vi "Coeficientes do polinômio.vi"(1 "R":dbl=0.06009682, 2 "Infos para processamento":T1={"Diâmetro do furo [mm]"=1.4, "Diâmetro da linha média [mm]"=5.0, "IncF"=0.2, "Módulo de elasticidade [GPa]"=207.0, "Módulo de Poisson"=0.3, "Tipo de roseta utilizada"=enum."Tipo A", "Método de análise"=enum."Simplificado 2008", "Pfinal"=0.3, "Parar auto."=TRUE}, 3 "Resultados":dbl[][](array[numeric])) -> (0 "Coeficientes":dbl[][](array[numeric]))   [LabVIEW 2016]
uses:
  Controles/Infos para processamento.ctl
  <vilib>/gmath/interp.llb/Interpolate 2D (1d xi,yi).vi
  <vilib>/gmath/NI_Gmath.lvlib
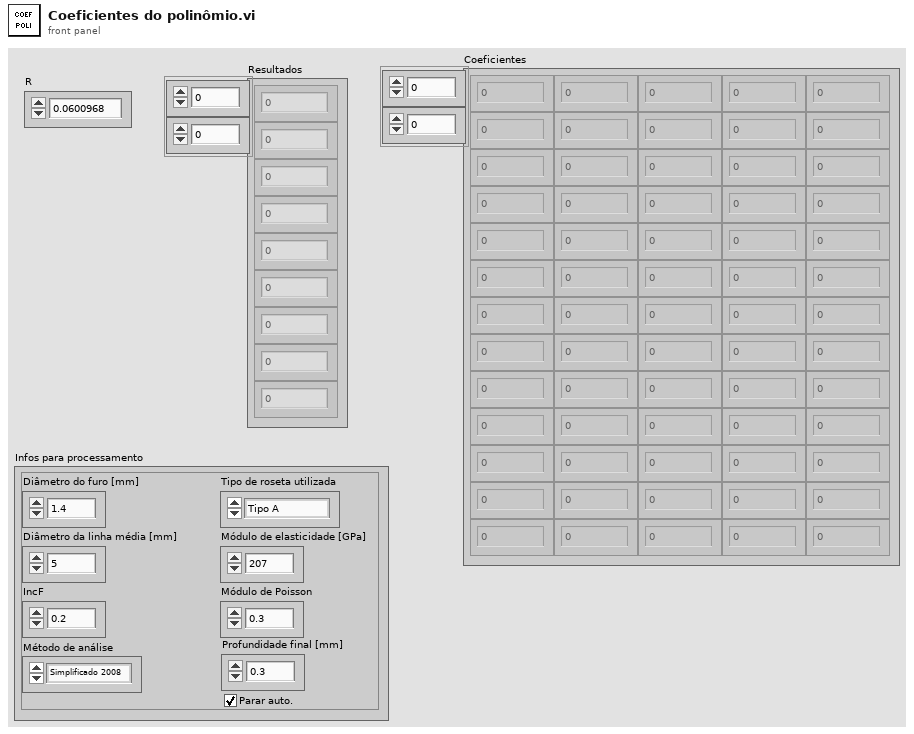
[diagram p1: front panel]
types:
  T1 = typedef "Infos para processamento.ctl" = cluster{"Diâmetro do furo [mm]":dbl, "Diâmetro da linha média [mm]":dbl, "IncF":dbl, "Módulo de elasticidade [GPa]":dbl, "Módulo de Poisson":dbl, "Tipo de roseta utilizada":enum16{"Tipo A", "Tipo B", "Tipo C"}, "Método de análise":enum16{"Não uniforme 2013", "Simplificado 2013", "Simplificado 2008"}, "Pfinal":dbl, "Parar auto.":bool}
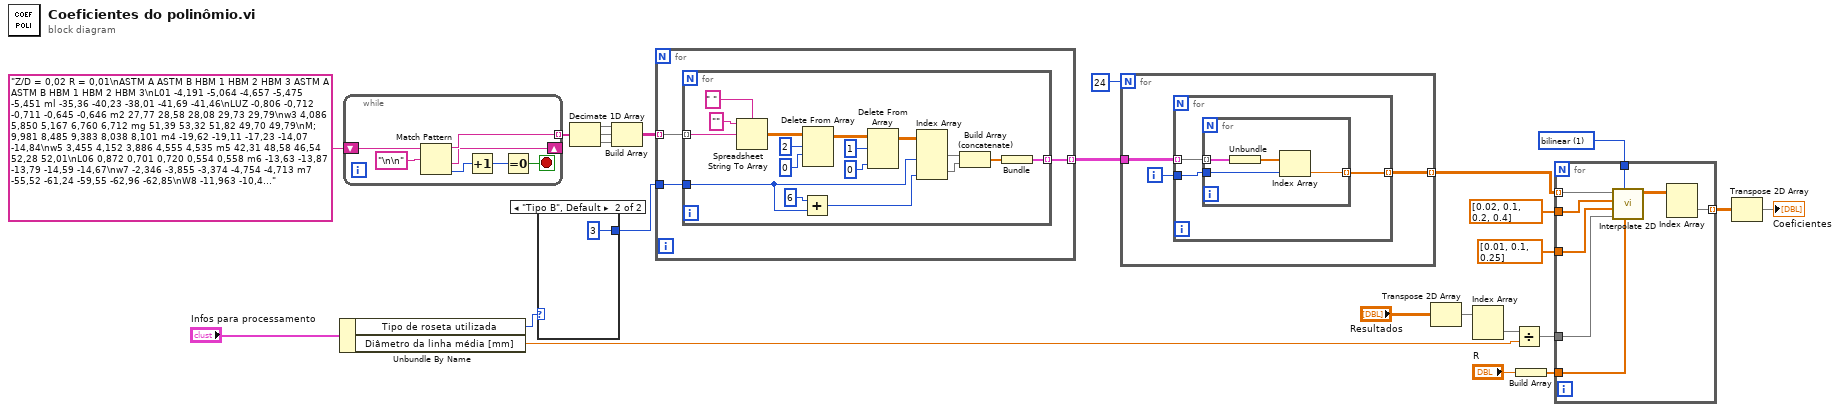
[diagram p0: block diagram]
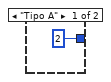
[diagram p2: hidden frame]
diagram:
  w1 = 1 items=["nearest", "bilinear", "bicubic", "bicubic spline"] ("method")
  n1 = Unbundle By Name("Infos para processamento") -> ("Tipo de roseta utilizada"=w23:enum16{"Tipo A", "Tipo B", "Tipo C"}, "Diâmetro da linha média [mm]"=w8:dbl)
  n2 = while {
    shift-right: [w25] -> _
    shift-left: "Z/D = 0,02 R = 0,01\nASTM A ASTM B HBM 1 HBM 2 HBM 3 ASTM A ASTM B HBM 1 HBM 2 HBM 3\nL01 -4,191 -5,064 -4,657 -5,475 -5,451 ml -35,36 -40,23 -38,01 -41,69 -41,46\nLUZ -0,806 -0,712 -0,711 -0,645 -0,646 m2 27,77 28,58 28,08 29,73 29,79\nw3 4,086 5,850 5,167 6,760 6,712 mg 51,39 53,32 51,82 49,70 49,79\nM; 9,981 8,485 9,383 8,038 8,101 m4 -19,62 -19,11 -17,23 -14,07 -14,84\nw5 3,455 4,152 3,886 4,555 4,535 m5 42,31 48,58 46,54 52,28 52,01\nL06 0,872 0,701 0,720 0,554 0,558 m6 -13,63 -13,87 -13,79 -14,59 -14,67\nw7 -2,346 -3,855 -3,374 -4,754 -4,713 m7 -55,52 -61,24 -59,55 -62,96 -62,85\nW8 -11,963 -10,454 -11,265 -9,883 -9,943 mg 3,10 4,60 2,90 2,60 3,17\nLU9 -0,525 -0,647 -0,609 -0,725 -0,722 mg -11,18 -12,43 -12,11 -13,29 -13,23\nW10 -0,203 -0,143 -0,153 -0,093 -0,095 mm -1,81 -1,59 -1,65 -1,35 -1,34\nwll -0,175 0,135 0,048 0,326 0,318 mm 12,06 13,46 13,18 14,19 14,15\nW12 4,390 3,993 4,198 3,836 3,850 ”112 17,86 16,93 17,49 16,92 16,83\n\nZ/D = 0,02 R = 0,1\nASTM A ASTM B HBM 1 HBM 2 HBM 3 ASTM A ASTM B HBM 1 HBM 2 HBM 3\nL01 -2,949 -3,650 -3,366 -4,011 -3,990 ml -31,83 -35,63 -34,29 -37,08 -36,69\nLUZ -0,760 -0,705 -0,713 -0,663 -0,664 mg 26,79 26,87 26,37 27,38 27,44\nw3 2,838 4,275 3,760 5,043 5,004 mg 48,54 49,43 48,85 46,24 46,19\nM; 9,695 8,415 9,226 8,054 8,112 m4 -16,90 -15,73 -13,94 -10,45 -11,25\nw5 2,363 2,931 2,748 3,276 3,259 m5 39,47 44,80 43,46 48,30 47,91\nL06 0,806 0,679 0,704 0,571 0,574 m6 -12,98 -12,69 -12,59 -12,91 -12,98\nw7 -1,398 -2,646 -2,282 -3,402 -3,368 m7 -53,71 -58,33 -57,43 -59,99 -59,79\nwg -11,475 -10,159 -10,901 -9,687 -9,742 mg -0,01 0,87 -0,76 -1,50 -0,91\nwg -0,293 -0,396 -0,370 -0,463 -0,460 mg -10,83 -11,90 -11,72 -12,72 -12,64\nW10 -0,188 -0,138 -0,149 -0,098 -0,099 mm -2,04 -1,90 -1,98 -1,75 -1,74\nwu -0,328 -0,063 -0,131 0,100 0,093 mm 12,06 13,24 13,11 13,93 13,88\nwlz 4,110 3,753 3,944 3,617 3,631 mm 19,02 18,17 18,75 18,24 18,14\n\nZ/D = 0,02 R = 0,25\nASTM A ASTM B HBM 1 HBM 2 HBM 3 ASTM A ASTM B HBM 1 HBM 2 HBM 3\nwl -1,609 -2,125 -1,932 -2,403 -2,387 ml -27,32 -29,77 -29,20 -30,90 -30,46\nwz -0,651 -0,607 -0,620 -0,568 -0,567 mg 26,45 25,49 25,40 25,48 25,41\nW3 1,434 2,512 2,135 3,098 3,067 mg 44,78 44,48 44,71 41,31 41,05\nw4 9,319 8,249 8,946 7,954 8,003 m4 -12,18 -10,36 -8,85 -4,74 -5,89\nw5 1,211 1,644 1,514 1,910 1,897 m5 36,34 40,55 39,77 43,62 43,15\nw6 0,687 0,585 0,610 0,500 0,501 m6 -12,77 -11,66 -11,89 -11,48 -11,44\nw7 -0,381 -1,348 -1,070 -1,933 -1,906 m7 -52,00 -55,45 -55,20 -56,72 -56,34\nwg -10,836 -9,713 -10,365 -9,326 -9,373 mg -5,92 -5,61 -7,04 -8,45 -7,57\nwg -0,070 -0,155 -0,134 -0,209 -0,207 mg -10,68 -11,58 -11,49 -12,31 -12,21\nW10 -0,167 -0,125 -0,134 -0,092 -0,093 mm -2,34 -2,34 -2,35 -2,25 -2,27\nwu -0,451 -0,234 -0,290 -0,101 -0,107 mm 12,44 13,42 13,41 14,03 13,95\nwlz 3,742 3,427 3,599 3,311 3,323 mm 21,46 20,66 21,23 20,80 20,64\n\nZ/D = 0,1 R = 0,01\nASTM A ASTM B HBM 1 HBM 2 HBM 3 ASTM A ASTM B HBM 1 HBM 2 HBM 3\nwl -4,322 -5,171 -4,957 -5,773 -5,755 ml 5,73 1,23 4,02 -0,33 -0,23\nwz -1,396 -1,294 -1,304 -1,005 -1,014 mg 15,08 17,79 16,30 20,62 20,47\nW3 3,464 5,118 4,658 6,121 6,090 mg -11,55 -3,29 -7,58 -0,38 -0,55\nw4 2,804 1,894 2,250 1,273 1,302 m4 -3,59 -8,92 -7,17 -13,47 -13,28\nw5 4,010 4,642 4,528 5,134 5,120 m5 -7,93 -4,64 -6,31 -3,54 -3,60\nw6 1,765 1,612 1,648 1,295 1,306 m6 -8,40 -10,28 -9,34 -12,58 -12,47\nw7 -3,079 -4,462 -4,124 -5,340 -5,313 m7 16,34 9,47 12,40 6,90 7,01\nwg -4,039 -3,130 -3,449 -2,463 -2,493 mg 1,37 6,31 4,79 10,45 10,29\nwg -0,872 -0,947 -0,946 -1,013 -1,011 mg 1,83 1,16 1,43 0,91 0,92\nW10 -0,487 -0,433 -0,451 -0,349 -0,352 mm 0,09 0,41 0,25 0,87 0,85\nwu 0,563 0,804 0,752 0,952 0,948 mm -4,74 -3,24 -3,78 -2,63 -2,65\nwlz 1,659 1,431 1,514 1,271 1,278 mm 6,39 5,27 5,62 4,37 4,40\n\nZ/D = 0,1 R = 0,1\nASTM A ASTM B HBM 1 HBM 2 HBM 3 ASTM A ASTM B HBM 1 HBM 2 HBM 3\nwl -2,006 -2,664 -2,447 -3,123 -3,107 ml -2,36 -5,38 -2,94 -6,17 -6,09\nwz -1,271 -1,253 -1,262 -1,069 -1,079 mg 9,61 11,71 10,42 14,40 14,22\nW3 1,541 2,826 2,425 3,600 3,573 mg -2,94 3,57 -0,21 5,65 5,50\nw4 2,446 1,767 2,056 1,324 1,349 m4 0,90 -3,91 -2,30 -8,23 -8,02\nw5 1,967 2,481 2,343 2,868 2,855 m5 -1,10 1,08 -0,39 1,62 1,58\nw6 1,467 1,394 1,425 1,191 1,201 m6 -4,33 -5,75 -4,94 -7,84 -7,71\nw7 -1,400 -2,500 -2,193 -3,188 -3,165 m7 9,20 3,69 6,28 1,73 1,84\nw8 -3,409 -2,724 -2,981 -2,248 -2,272 mg -2,23 2,23 0,83 6,04 5,87\nwg -0,417 -0,487 -0,473 -0,542 -0,541 mg 0,59 0,09 0,35 -0,08 -0,07\nW10 -0,381 -0,345 -0,360 -0,288 -0,291 mm -0,67 -0,41 -0,56 0,00 -0,02\nwu 0,201 0,402 0,349 0,522 0,518 mm -3,41 -2,13 -2,63 -1,62 -1,65\nwlz 1,374 1,197 1,265 1,081 1,087 mm 6,93 5,89 6,22 5,07 5,11\n\nZ/D = 0,1 R = 0,25\nASTM A ASTM B HBM 1 HBM 2 HBM 3 ASTM A ASTM B HBM 1 HBM 2 HBM 3\nwl -1,541 -1,984 -1,820 -2,291 -2,278 ml -1,46 -3,94 -1,55 -4,16 -4,09\nwz -0,903 -0,942 -0,935 -0,861 -0,866 mg 7,60 9,26 8,13 11,52 11,37\nW3 1,190 2,082 1,791 2,617 2,595 mg -4,05 1,68 -1,85 3,24 3,10\nw4 1,891 1,435 1,639 1,162 1,179 m4 3,28 -1,16 0,33 -5,05 -4,86\nw5 1,436 1,795 1,684 2,059 2,049 m5 -2,10 -0,35 -1,83 -0,27 -0,31\nw6 1,012 1,002 1,014 0,903 0,908 m6 -3,06 -4,17 -3,45 -5,88 -5,77\nw7 -1,008 -1,787 -1,559 -2,268 -2,249 m7 10,47 5,64 8,07 4,15 4,25\nwg -2,595 -2,128 -2,311 -1,830 -1,846 mg -4,19 -0,06 -1,39 3,32 3,16\nwg -0,274 -0,328 -0,314 -0,368 -0,366 mg 0,97 0,54 0,80 0,44 0,45\nW10 -0,255 -0,236 -0,245 -0,204 -0,206 mm -0,88 -0,67 -0,80 -0,33 -0,35\nwu 0,107 0,256 0,214 0,342 0,339 mm -3,85 -2,69 -3,17 -2,26 -2,28\nwlz 1,035 0,911 0,960 0,835 0,839 mm 7,23 6,25 6,57 5,51 5,55\n\nZ/D = 0,2 R = 0,01\nASTM A ASTM B HBM 1 HBM 2 HBM 3 ASTM A ASTM B HBM 1 HBM 2 HBM 3\nL01 -3,758 -4,157 -4,224 -4,676 -4,659 ml -30,41 -34,62 -35,17 -41,37 -41,15\nLUZ -0,022 -0,007 -0,129 -0,024 -0,032 mg 26,25 25,88 25,07 24,06 24,07\nW3 3,215 4,350 4,084 5,233 5,199 mg 11,41 20,15 18,25 30,99 30,57\nW4 3,770 3,136 3,406 2,691 2,715 m4 4,03 0,45 2,80 -3,05 -2,83\nMg 3,523 3,753 3,858 4,098 4,087 m5 15,86 17,31 18,35 20,52 20,44\nLU6 0,502 0,459 0,555 0,406 0,415 m6 -18,71 -18,24 -17,85 -17,07 -17,08\nw7 -3,424 -4,393 -4,201 -5,123 -5,097 m7 -0,08 -6,11 -4,98 -12,97 -12,71\nW8 -4,583 -3,867 -4,135 -3,352 -3,377 mg -3,24 0,73 -1,31 4,24 4,05\nwg -0,862 -0,852 -0,888 -0,872 -0,872 mg -1,73 -1,98 -2,18 -2,45 -2,44\nW10 -0,180 -0,150 -0,174 -0,116 -0,118 mm 2,99 2,80 2,76 2,58 2,58\nW11 0,978 1,142 1,116 1,254 1,250 mm -2,61 -1,22 -1,48 0,08 0,04\nW12 1,579 1,379 1,452 1,242 1,248 mm 5,06 4,08 4,51 3,27 3,31\n\nZ/D = 0,2 R = 0,1\nASTM A ASTM B HBM 1 HBM 2 HBM 3 ASTM A ASTM B HBM 1 HBM 2 HBM 3\nL01 -2,317 -2,682 -2,743 -3,073 -3,062 ml -5,92 -9,62 -10,71 -14,86 -14,71\nLUZ -0,027 -0,112 -0,197 -0,177 -0,184 mg 16,88 17,16 16,18 16,33 16,28\nW3 1,752 2,747 2,525 3,420 3,396 mg -9,21 -0,59 -2,14 8,38 8,05\nW4 2,839 2,371 2,575 2,052 2,071 m4 7,39 2,80 5,30 -1,23 -0,98\nMg 2,202 2,470 2,545 2,757 2,750 m5 -3,11 -1,48 -0,20 1,06 1,01\nwe 0,339 0,385 0,452 0,395 0,402 m6 -11,79 -11,71 -11,18 -11,16 -11,12\nw7 -2,050 -2,939 -2,764 -3,526 -3,506 m7 16,56 10,04 11,06 4,09 4,30\nW8 -3,511 -2,980 -3,184 -2,613 -2,633 mg -6,60 -1,98 -4,11 1,80 1,59\nw9 -0,539 -0,557 -0,582 -0,584 -0,584 m9 2,00 1,64 1,42 1,22 1,23\nW10 -0,112 -0,102 -0,120 -0,086 -0,088 mm 1,68 1,57 1,50 1,45 1,45\nW11 0,636 0,800 0,771 0,898 0,895 mm -5,95 -4,39 -4,65 -3,18 -3,22\nW12 1,232 1,079 1,135 0,979 0,984 mm 5,72 4,61 5,06 3,76 3,80\n\nZ/D = 0,2 R = 0,25\nASTM A ASTM B HBM 1 HBM 2 HBM 3 ASTM A ASTM B HBM 1 HBM 2 HBM 3\nL01 -1,101 -1,418 -1,428 -1,726 -1,717 ml -8,58 -13,09 -13,92 -19,11 -18,94\nLUZ -0,125 -0,198 -0,271 -0,272 -0,276 mg 14,80 14,50 13,62 13,36 13,35\nW3 0,770 1,552 1,359 2,059 2,041 mg -4,55 4,70 3,16 14,04 13,71\nW4 2,173 1,836 1,982 1,627 1,639 m4 8,01 4,15 6,25 0,97 1,17\nMg 1,108 1,360 1,382 1,599 1,593 m5 0,10 2,45 3,50 5,73 5,67\nLU6 0,283 0,328 0,388 0,366 0,369 m6 -10,53 -10,02 -9,52 -9,17 -9,16\nw7 -1,059 -1,767 -1,609 -2,217 -2,201 m7 12,03 4,99 6,02 -1,34 -1,12\nW8 -2,632 -2,257 -2,403 -2,020 -2,033 mg -7,34 -3,39 -5,21 -0,36 -0,54\nwg -0,274 -0,304 -0,314 -0,334 -0,334 mg 1,29 0,79 0,61 0,22 0,23\nW10 -0,071 -0,066 -0,082 -0,061 -0,062 mm 1,45 1,27 1,19 1,09 1,09\nW11 0,359 0,497 0,469 0,577 0,575 mm -4,99 -3,33 -3,59 -2,05 -2,09\nW12 0,908 0,800 0,840 0,734 0,737 mm 5,81 4,83 5,23 4,12 4,16\n\nZ/D = 0,4 R = 0,01\nASTM A ASTM B HBM 1 HBM 2 HBM 3 ASTM A ASTM B HBM 1 HBM 2 HBM 3\nL01 -1,579 -1,604 -1,750 -1,567 -1,568 ml 6,11 6,91 6,52 9,38 9,30\nLUZ 1,636 1,847 1,753 1,704 1,706 mg 16,56 22,63 22,18 20,11 20,30\nW3 0,348 0,783 0,690 1,246 1,223 mg -20,14 -25,83 -26,06 -23,21 -23,49\nW4 4,662 4,017 4,355 3,619 3,644 m4 11,99 10,26 11,97 7,10 7,31\nMg 1,950 1,924 2,020 1,786 1,788 m5 -12,47 -12,63 -12,58 -15,59 -15,51\nLU6 -0,569 -0,733 -0,706 -0,677 -0,678 m6 -8,93 -14,37 -14,04 -12,89 -13,02\nw7 -1,383 -1,904 -1,784 -2,324 -2,303 m7 21,64 25,41 25,84 24,22 24,41\nW8 -5,469 -4,673 -4,997 -4,162 -4,188 mg -11,04 -8,47 -9,97 -5,37 -5,56\nwg -0,841 -0,778 -0,803 -0,695 -0,697 mg 2,93 2,64 2,74 3,15 3,14\nW10 -0,042 0,013 0,008 0,032 0,031 mm 1,43 2,42 2,38 2,10 2,12\nW11 0,965 1,060 1,039 1,119 1,116 mm -5,88 -6,02 -6,26 -5,57 -5,61\nW12 1,846 1,602 1,686 1,445 1,452 ”112 5,81 5,07 5,40 4,35 4,39\n\nZ/D = 0,4 R = 0,1\nASTM A ASTM B HBM 1 HBM 2 HBM 3 ASTM A ASTM B HBM 1 HBM 2 HBM 3\nL01 0,494 0,357 0,196 0,295 0,297 ml 13,01 12,18 11,60 14,90 14,84\nLUZ 1,539 1,592 1,521 1,396 1,398 mg 17,08 22,05 22,02 18,90 19,07\nW3 -1,437 -0,836 -0,929 -0,354 -0,375 mg -26,95 -28,67 -29,66 -25,81 -26,10\nW4 3,280 2,759 3,033 2,474 2,494 m4 10,26 7,39 9,39 4,56 4,77\nMg -0,015 0,090 0,190 0,067 0,067 m5 -16,43 -15,55 -15,26 -18,63 -18,56\nw6 -0,746 -0,773 -0,756 -0,654 -0,655 m6 -10,54 -14,76 -14,83 -12,58 -12,70\nw7 0,442 -0,202 -0,084 -0,637 -0,619 m7 26,63 27,29 28,27 25,68 25,88\nw8 -3,933 -3,312 -3,572 -2,946 -2,966 m8 -9,61 -6,31 -8,00 -3,50 -3,68\nw9 -0,279 -0,264 -0,285 -0,220 -0,222 mg 3,69 3,27 3,31 3,83 3,81\nw10 0,053 0,076 0,073 0,076 0,075 m10 1,76 2,48 2,52 2,01 2,03\nw11 0,401 0,530 0,507 0,602 0,599 m11 -6,78 -6,38 -6,70 -5,85 -5,89\nw12 1,361 1,173 1,239 1,058 1,064 m12 5,37 4,51 4,87 3,84 3,88\n\nZ/D = 0,4 R = 0,25\nASTM A ASTM B HBM 1 HBM 2 HBM 3 ASTM A ASTM B HBM 1 HBM 2 HBM 3\nw1 0,773 0,575 0,432 0,411 0,413 m1 8,74 6,15 5,40 6,75 6,73\nw2 1,015 1,022 0,954 0,841 0,843 m2 14,63 19,02 18,99 15,93 16,09\nw3 -1,499 -0,927 -0,996 -0,462 -0,478 mg -20,56 -19,96 -20,98 -15,58 -15,88\nw4 2,323 1,961 2,161 1,782 1,795 m4 10,59 8,00 9,88 5,81 5,99\nw5 -0,470 -0,292 -0,206 -0,200 -0,201 m5 -13,21 -10,95 -10,55 -12,25 -12,20\nw6 -0,517 -0,506 -0,482 -0,382 -0,384 m6 -8,76 -12,47 -12,55 -10,29 -10,41\nw7 0,833 0,238 0,330 -0,182 -0,167 m7 22,23 21,08 22,09 18,11 18,32\nw8 -2,764 -2,338 -2,526 -2,104 -2,118 m8 -10,38 -7,35 -8,96 -5,04 -5,20\nw9 -0,054 -0,072 -0,087 -0,066 -0,067 mg 3,31 2,65 2,67 2,86 2,85\nw10 0,053 0,063 0,059 0,055 0,055 m10 1,34 1,96 2,01 1,50 1,52\nw11 0,131 0,258 0,238 0,336 0,333 m11 -6,19 -5,46 -5,78 -4,66 -4,71\nw12 0,953 0,823 0,871 0,747 0,751 m12 5,54 4,72 5,08 4,15 4,18" ("text") -> [w30]
    tunnel: [w29] -> w22 mode=indexing
    stop <- w26 stop-if-true
    n3 = Match Pattern(string=w30, regular expression="\n\n") -> (before substring=w29:string, after substring=w25:string, offset past match=w28:i32)  [unwired: 1 in, 1 out]
    n4 = Increment(x=w28) -> (x+1=w27:i32)
    n5 = Equal To 0?(x=w27) -> (x = 0?=w26:bool)
  }
  n6 = case shown="\"Tipo B\", Default" w23 {
    tunnel: [2 3] -> w17
    frame "Tipo A" {
    }
    frame "Tipo B", Default {
    }
  }
  n7 = Decimate 1D Array(w22) -> (w19:string[], w20:string[], w21:string[])
  n8 = Build Array(w19, w20, w21) -> (w18:string[][])
  n9 = for {
    tunnel: w18 -> [w36] mode=indexing
    tunnel: w17 -> [w35]
    tunnel: [w34] -> w16 mode=indexing
    n10 = for {
      tunnel: w36 -> [w51] mode=indexing
      tunnel: w35 -> [w42]
      tunnel: [w37] -> w34 mode=indexing
      n11 = Spreadsheet String To Array(delimiter (Tab)=" ", format string="", spreadsheet string=w51) -> (array=w50:dbl[][])  [unwired: 1 in]
      n12 = Add(x=6 ("index (row)"), y=w42) -> (x+y=w41:i32)
      n13 = Delete From Array(array=w50, length=2, index (row)=0) -> (array with subset deleted=w46:dbl[][])  [unwired: 1 in, 1 out]
      n14 = Delete From Array(array=w46, length=1, index (col)=0 ("index (row)")) -> (array with subset deleted=w44:dbl[][])  [unwired: 1 in, 1 out]
      n15 = Index Array(array=w44, index (col) #1=w42, index (col) #2=w41) -> (element #1=w39:dbl[], element #2=w40:dbl[])  [unwired: 2 in]
      n16 = Build Array (concatenate)(w39, w40) -> (w38:dbl[])
      n17 = Bundle(w38) -> (w37:cluster{dbl[]})  [unwired: 1 in]
    }
  }
  n18 = for {
    N: 24 -> [_]
    tunnel: w16 -> [w56]
    tunnel: [w54] -> w14 mode=indexing
    i -> [w55]
    n19 = for {
      tunnel: w56 -> [w59] mode=indexing
      tunnel: w55 -> [w58]
      tunnel: [w57] -> w54 mode=indexing
      n20 = for {
        tunnel: w59 -> [w63] mode=indexing
        tunnel: w58 -> [w61]
        tunnel: [w60] -> w57 mode=indexing
        n21 = Unbundle(w63) -> (w62:dbl[])
        n22 = Index Array(array=w62, index=w61) -> (element=w60:dbl)
      }
    }
  }
  n23 = Transpose 2D Array(2D array="Resultados") -> (transposed array=w12:dbl[][])
  n24 = Index Array(array=w12) -> (element=w9:dbl[])  [unwired: 2 in]
  n25 = Divide(x=w9, y=w8) -> (x/y=w7:dbl[])
  n26 = Build Array("R") -> (w5:dbl[])
  n27 = for {
    tunnel: w14 -> [w71] mode=indexing
    tunnel: dbl[] [0.02, 0.1, 0.2, 0.4] ("X") -> [w70]
    tunnel: dbl[] [0.01, 0.1, 0.25] ("Y") -> [w69]
    tunnel: w7 -> [w68]
    tunnel: w5 -> [w67]
    tunnel: [w65] -> w4 mode=indexing
    tunnel: w1 -> [w64]
    n28 = call-poly <vilib>:"Interpolate 2D.vi"("yi"=w67, "method"=w64, "xi"=w68, "Y"=w69, "X"=w70, "Z"=w71) -> ("zi"=w66:dbl[][])  [unwired: 2 in, 3 out]
    n29 = Index Array(array=w66) -> (element=w65:dbl[])  [unwired: 2 in]
  }
  n30 = Transpose 2D Array(2D array=w4) -> (transposed array=→"Coeficientes":dbl[][])
